vi "Add Default Enum.vi"(6 "Hdr Name":T1, 8 "error in (no error)":errorcluster, 9 "Enum Values":u16[](array[numeric]), 11 "Current in":refnum<class "Current.lvclass">) -> (0 "error out":errorcluster, 3 "Current out":refnum<class "Current.lvclass">)   [LabVIEW 2012, in "Measurement Channels.lvlib" / "Current.lvclass"]
uses:
  Current.lvclass
  Common/Controls/HeaderNames.ctl
  Current.lvclass/Current.ctl
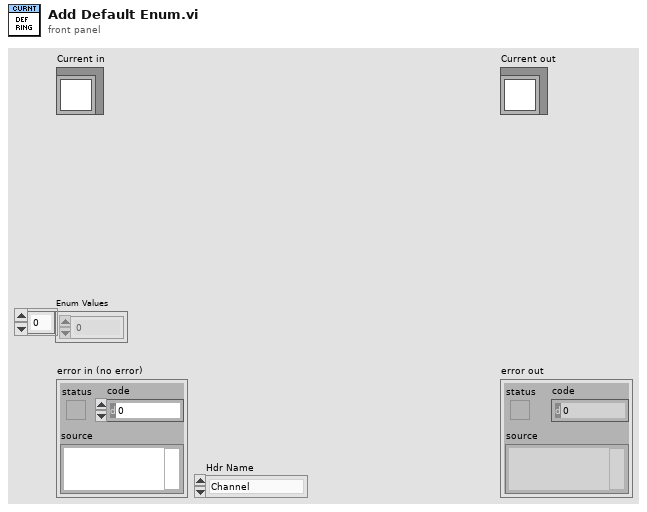
[diagram p1: front panel]
types:
  T1 = typedef "HeaderNames.ctl" = enum16{"Channel", "Device", "Spacer", "Description", "MB", "Range", "Terminal", "Coupling", "Thresh (V)", "Pulse/Rev", "Slope", "Min EU", "Min RPM", "mV/EU", "Iex", "Temp Units", "Type", "CJC Src", "CJC Val", "Ro", "Wire Cfg", "Strain Mode", "Vex", "Bridge Type", "GF", "Gauge Res", "Poisson", "Lead Res", "Init Strain", "GAF", "Scale", "Offset", "Unit (EU)", "dB?", "dB Ref", "Cal Mag", "Cal Units", "Max Temp", "Min Temp", "Max Strain", "Min Strain"}
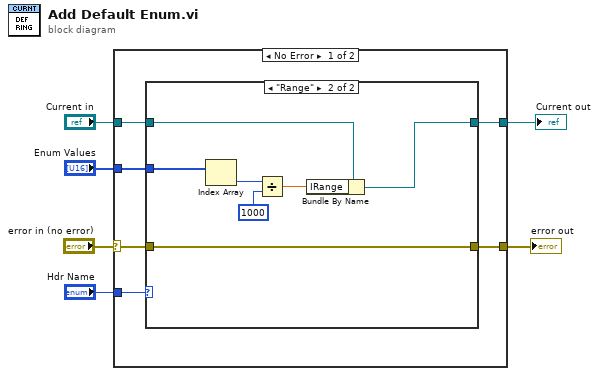
[diagram p0: block diagram]
diagram:
  n1 = case shown="No Error" "error in (no error)" {
    selector: "error in (no error)" -> [w7 w23]
    tunnel: "Current in" -> [w12 w22]
    tunnel: "Enum Values" -> [w11 _]
    tunnel: [w10 w22] -> w4
    tunnel: "Hdr Name" -> [w9 _]
    tunnel: [w8 w23] -> w2
    frame No Error {
      n2 = case shown="\"Range\"" w9 {
        tunnel: w12 -> [w14 w21]
        tunnel: w11 -> [_ w18]
        tunnel: [w14 w16] -> w10
        tunnel: w7 -> [w13 w15]
        tunnel: [w13 w15] -> w8
        frame Default {
        }
        frame "Range" {
          n3 = Index Array(array=w18) -> (element=w20:u16)  [unwired: 1 in]
          n4 = Divide(x=w20, y=1000) -> (x/y=w17:dbl)
          n5 = Bundle By Name(cluster=w21, "IRange"=w17) -> (w16:refnum<class "Current.lvclass">)
        }
      }
    }
    frame Error {
    }
  }
  "error out" <- w2
  "Current out" <- w4
